vi "Preview.vi"(8 "error in (no error)":errorcluster, 9 "timeout in ms (-1)":i32=-1, 11 "Queue in":refnum<class "Queue.lvclass">) -> (0 "error out":errorcluster, 1 "timed out?":bool, 2 "Data":refnum<class "Data.lvclass">, 3 "Queue out":refnum<class "Queue.lvclass">)   [LabVIEW 2020, in "Data.lvlib" / "Queue.lvclass"]
doc: "Preview the front most data element."
uses:
  Queue.lvclass
  Data.lvclass
  Queue.lvclass/Queue.ctl
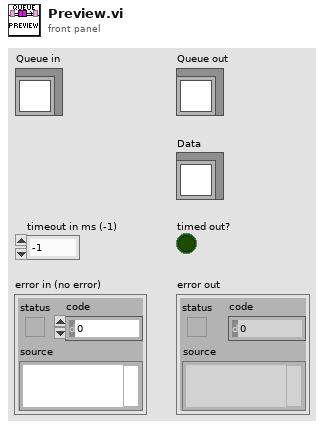
[diagram p1: front panel]
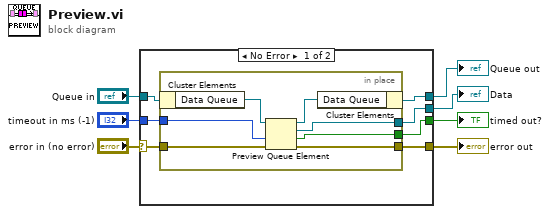
[diagram p0: block diagram]
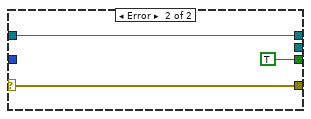
[diagram p2: hidden frame]
diagram:
  n1 = case shown="No Error" "error in (no error)" {
    selector: "error in (no error)" -> [w11 w24]
    tunnel: [w10 w24] -> w6
    tunnel: [w13 w23] -> w4
    tunnel: "Queue in" -> [w14 w23]
    tunnel: "timeout in ms (-1)" -> [w12 _]
    tunnel: [w9 TRUE ("timed out?")] -> w2
    tunnel: [w8 _] -> w1
    frame No Error {
      n2 = in-place {
        in-place-border: w12 -> [w16]
        in-place-border: w11 -> [w15]
        in-place-border: [w19] -> w10
        in-place-border: [w18] -> w9
        in-place-border: [w17] -> w8
        n3 = in-place-cluster #1(w14) -> ("Data Queue"=w21:refnum<queue>)
        n4 = Preview Queue Element(queue=w21, timeout in ms (-1)=w16, error in (no error)=w15) -> (queue out=w20:refnum<queue>, element=w17:refnum<class "Data.lvclass">, timed out?=w18:bool, error out=w19:errorcluster)
        n5 = in-place-cluster #1("Data Queue"=w20) -> (w13:refnum<class "Queue.lvclass">)
      }
    }
    frame Error {
    }
  }
  "error out" <- w6
  "Queue out" <- w4
  "Data" <- w1
  "timed out?" <- w2
